vi "Move To Impl.vi"(8 "error in (no error)":errorcluster, 9 "Index":u16, 10 "Area":enum16{"Home", "Well", "Wash Port"}(ring), 11 "Autosampler in":refnum<class "Autosampler.lvclass">) -> (0 "error out":errorcluster, 3 "Autosampler out":refnum<class "Autosampler.lvclass">)   [LabVIEW 2023, in "Autosampler.lvlib" / "Autosampler.lvclass"]
uses:
  Autosampler.lvclass
  Autosampler.lvclass/Autosampler.ctl
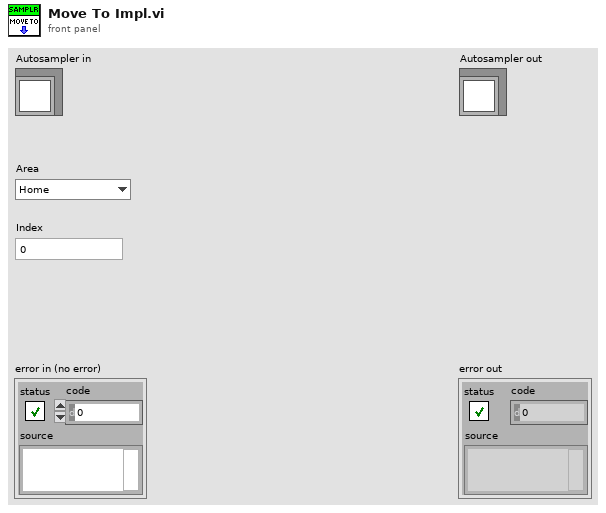
[diagram p1: front panel]
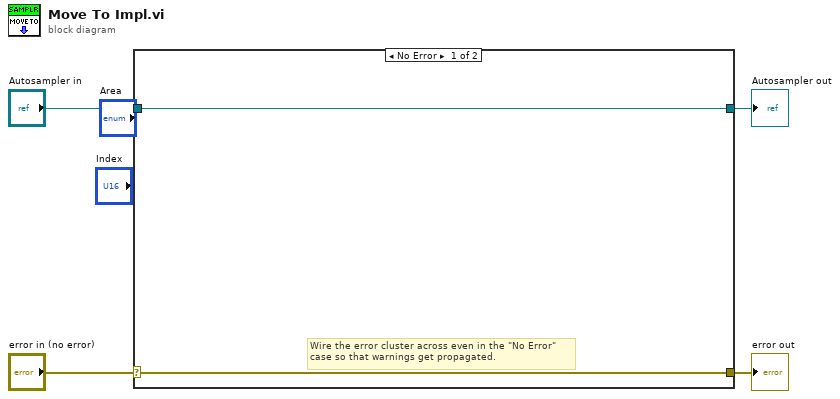
[diagram p0: block diagram]
diagram:
  n1 = case shown="No Error" "error in (no error)" {
    selector: "error in (no error)" -> [w5 w8]
    tunnel: [w5 w8] -> w3
    tunnel: [w6 w7] -> w1
    tunnel: "Autosampler in" -> [w6 w7]
    frame No Error {
      # "Wire the error cluster across even in the \"No Error\"\ncase so that warnings get propagated."
    }
    frame Error {
    }
  }
  "error out" <- w3
  "Autosampler out" <- w1
